vi "Read_Instr.vi"(8 "error in (no error)":errorcluster caption="entrée d'erreur (pas d'erreur)", 11 "Class Instrument Firebase en entrée":refnum<class "Class Instrument Firebase Altyor.lvclass">) -> (0 "error out":errorcluster caption="sortie d'erreur", 3 "Class Instrument Firebase en sortie":refnum<class "Class Instrument Firebase Altyor.lvclass">)   [LabVIEW 2020, in "Library Instrument & Equipement.lvlib" / "Library Instruments.lvlib" / "Class Instrument Firebase Altyor.lvclass"]
uses:
  Class Instrument Firebase Altyor.lvclass
  Class Instrument Firebase Altyor.lvclass/Class Instrument Firebase Altyor.ctl
  Instrument (Default)/Class Instrument (Default).lvclass
  Firebase/Source/Firebase Altyor/Firebase Altyor.lvclass
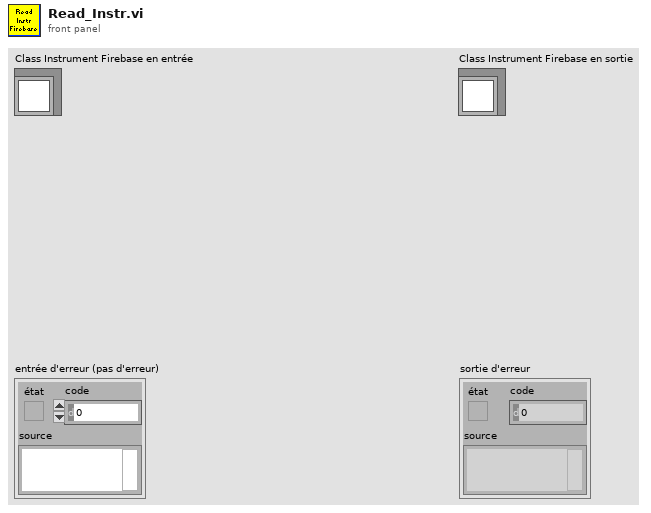
[diagram p1: front panel]
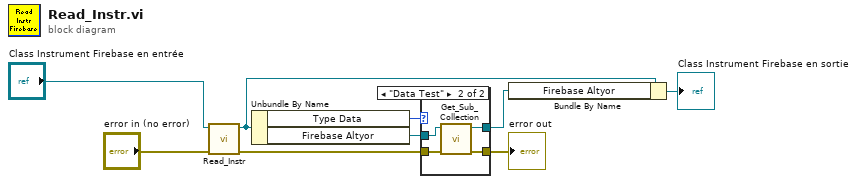
[diagram p0: block diagram]
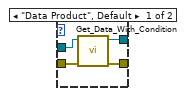
[diagram p2: hidden frame]
diagram:
  n1 = call-parent "Read_Instr.vi"("error in (no error)"="error in (no error)", "Class Instrument (Default) en entrée"="Class Instrument Firebase en entrée") -> ("error out"=w5:errorcluster, "Class Instrument (Default) en sortie"=w3:refnum<class "Class Instrument Firebase Altyor.lvclass">)  [unwired: 8 in]
  n2 = Unbundle By Name(w3) -> ("Type Data"=w7:enum16{"Data Product", "Data Test"}, "Firebase Altyor"=w6:refnum<class "Firebase Altyor.lvclass">)
  n3 = case shown="\"Data Test\"" w7 {
    tunnel: w5 -> [w13 w16]
    tunnel: [w11 w15] -> w4
    tunnel: w6 -> [w12 w17]
    tunnel: [w10 w14] -> w1
    frame "Data Product", Default {
      n4 = call-dynamic "Get_Data_With_Condition.vi"("error in (no error)"=w13, "Firebase Benches en entrée"=w12) -> ("error out"=w11:errorcluster, "Firebase Benches en sortie"=w10:refnum<class "Firebase Altyor.lvclass">)  [unwired: 8 in]
    }
    frame "Data Test" {
      n5 = call-dynamic "Get_Sub_Collection.vi"("error in (no error)"=w16, "Firebase Altyor en entrée"=w17) -> ("error out"=w15:errorcluster, "Firebase Altyor en sortie"=w14:refnum<class "Firebase Altyor.lvclass">)  [unwired: 8 in]
    }
  }
  "error out" <- w4
  n6 = Bundle By Name(cluster=w3, "Firebase Altyor"=w1) -> (→"Class Instrument Firebase en sortie":refnum<class "Class Instrument Firebase Altyor.lvclass">)
